vi "Send Telemetry.vi"(11 "stop":bool) -> ()   [LabVIEW 2013]
uses:
  Global Data.vi
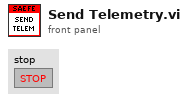
[diagram p1: front panel]
types:
  T1 = typedef "Telemetry.ctl" = cluster{"X Accel":dbl, "Y Accel":dbl, "Pack Current":dbl, "Pack Voltage":dbl, "SOC":dbl, "Avg. Throttle (%)":dbl, "Z Accel":dbl, "Throttle 1 (%)":dbl, "Throtttle 2 (%)":dbl, "Throttle 1 (V)":dbl, "Throttle 2 (V)":dbl, "Left Current (A)":dbl, "Right Current (A)":dbl, "Steering Wheel Angle (degrees)":dbl, "X Rotation Rate (mDegrees/s)":dbl, "Front Brake Pressure (psi)":dbl, "Rear Brake Pressure (psi)":dbl, "Computed Vehicle Speed (mph)":dbl, "BSPD Status":bool, "IMD Status":bool, "Motor Controller Enable":bool, "Left CEL":bool, "Right CEL":bool, "BMS Fault":bool, "Pre-Charge Finished":bool, "AIR Status":enum16{"Off", "Precharge", "On"}, "Y Rotation Rate (mDegrees/s)":dbl, "Z Rotation Rate (mDegrees/s)":dbl, "FPGA LED":bool, "Chassis Temperature":i16, "Throttles Consistent?":bool, "Throttles In Range?":bool, "TSMS Status":bool, "Latch Status":bool, "BMS Reduced Drive":bool, "BSPD Dash LED":bool, "IMD Dash LED":bool, "AMS Dash LED":bool, "Positive AIR Enable":bool}
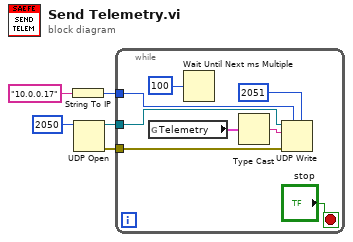
[diagram p0: block diagram]
diagram:
  n1 = String To IP(1:"10.0.0.17" ("net address")) -> (0:w1:u32)
  n2 = UDP Open(11:u16 2050 ("port")) -> (port=w5:refnum<k16>, 0:w4:errorcluster)  [unwired: 4 in, 1 out]
  n3 = while {
    tunnel: w5 -> [w11]
    tunnel: w4 -> [w10]
    tunnel: w1 -> [w7]
    stop <- "stop" stop-if-true
    n4 = global read "Global Data.vi" "Telemetry"() -> (w13:T1)
    n5 = Wait Until Next ms Multiple(millisecond multiple=u32 100 ("milliseconds to wait")) -> ()  [unwired: 1 out]
    n6 = Type Cast(x=w13) -> (*(type *) &x=w12:string)  [unwired: 1 in]
    n7 = UDP Write(address=w7, port or service name=u16 2051, connection ID=w11, data in=w12, 8:w10) -> ()  [unwired: 1 in, 2 out]
  }
